vi "RepIntIn.vi"(9 "Memory Size":i32, 11 "Input":dbl) -> (0 "output cluster":T1)   [LabVIEW 2010, in "KevLib01.lvlib"]
uses:
  KevLib01.lvlib
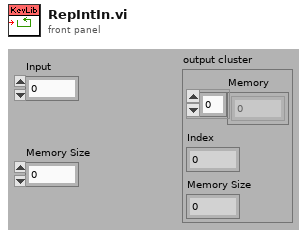
[diagram p1: front panel]
types:
  T1 = cluster{"Memory":dbl[], "Index":i32, "Memory Size":i32}
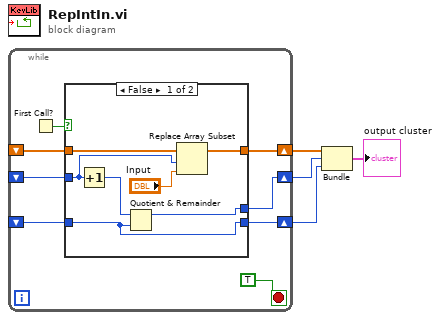
[diagram p0: block diagram]
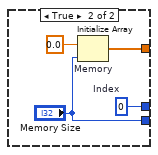
[diagram p2: hidden frame]
diagram:
  n1 = while {
    shift-right: [w11] -> w4
    shift-left: _ -> [w6]
    shift-right: [w10] -> w3
    shift-left: _ -> [w9]
    shift-right: [w8] -> w2
    shift-left: _ -> [w7]
    stop <- TRUE stop-if-true
    n2 = First Call?() -> (First Call?: T/F=w12:bool)
    n3 = case shown="False" w12 {
      tunnel: [w13 w22] -> w11
      tunnel: [w18 "Memory Size"] -> w10
      tunnel: w9 -> [w18 _]
      tunnel: [w17 w20] -> w8
      tunnel: w7 -> [w15 _]
      tunnel: w6 -> [w16 _]
      frame False {
        n4 = Increment(x=w15) -> (x+1=w19:i32)
        n5 = Quotient & Remainder(x=w19, y=w18) -> (x-y*floor(x/y)=w17:i32)  [unwired: 1 out]
        n6 = Replace Array Subset(array=w16, new element="Input", index=w15) -> (w13:dbl[])
      }
      frame True {
        w20 = 0  # Index
        n7 = Initialize Array "Memory"(0.0 ("element"), "Memory Size") -> (w22:dbl[])
      }
    }
  }
  n8 = Bundle(w4, "Index"=w2, "Memory Size"=w3) -> (→"output cluster":cluster{dbl[], "Index":i32, "Memory Size":i32})  [unwired: 1 out]
